vi "CLAD Exercise 4-1.vi"(8 "error in (no error)":errorcluster, 9 "Minimum Tempature":dbl, 10 "Maximum Tempature":dbl, 11 "Current Temp":dbl) -> (0 "error out":errorcluster, 1 "Warning":bool, 2 "Warning Text":string)   [LabVIEW 2014]
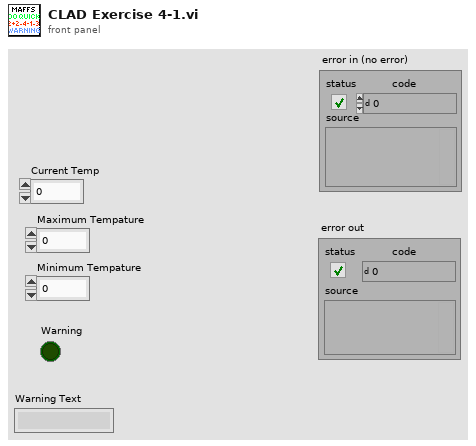
[diagram p1: front panel]
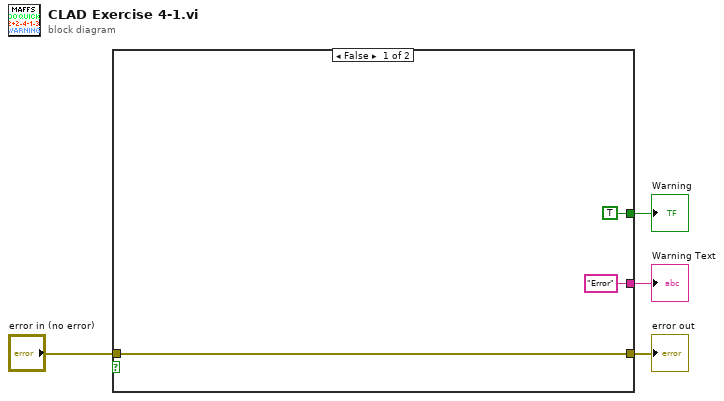
[diagram p0: block diagram]
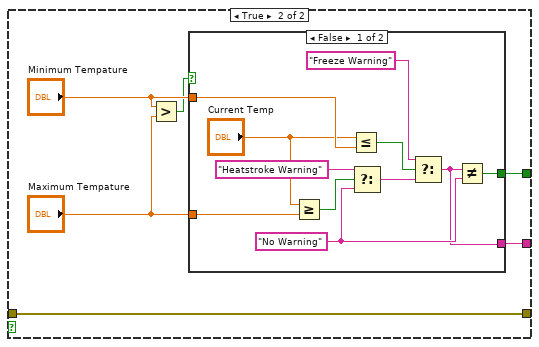
[diagram p2: hidden frame]
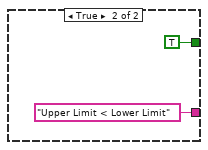
[diagram p3: hidden frame]
diagram:
  n1 = case shown="\"Eror\"" {
    selector: _ -> [_ _]
    tunnel: ["Error" w10] -> w3
    tunnel: [TRUE w9] -> w4
    tunnel: [w7 w8] -> w2
    tunnel: "error in (no error)" -> [w7 w8]
    frame False {
    }
    frame True {
      n2 = Greater?(x="Minimum Tempature", y="Maximum Tempature") -> (0:w11:bool)
      n3 = case shown="False" w11 {
        tunnel: "Minimum Tempature" -> [w24 _]
        tunnel: "Maximum Tempature" -> [w23 _]
        tunnel: [w15 TRUE] -> w9
        tunnel: [w14 "Upper Limit < Lower Limit"] -> w10
        frame False {
          w19 = "No Warning"
          n4 = Greater Or Equal?(x="Current Temp", y=w23) -> (x >= y?=w21:bool)
          n5 = Less Or Equal?(x="Current Temp", y=w24) -> (x <= y?=w18:bool)
          n6 = Select(t="Heatstroke Warning", s=w21, f=w19) -> (s? t:f=w16:string)
          n7 = Select(t="Freeze Warning", s=w18, f=w16) -> (s? t:f=w14:string)
          n8 = Not Equal?(x=w14, y=w19) -> (x != y?=w15:bool)
        }
        frame True {
        }
      }
    }
  }
  "error out" <- w2
  "Warning Text" <- w3
  "Warning" <- w4
